vi "Turn_off_lamp.vi"() -> ()   [LabVIEW 2011]
uses:
  <vilib>/Instr/_visa.llb/VISA Configure Serial Port (Instr).vi
panel:
  in  "VISA resource name":refnum<visa-resource-name>="COM4"
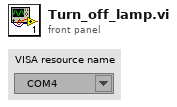
[diagram p1: front panel]
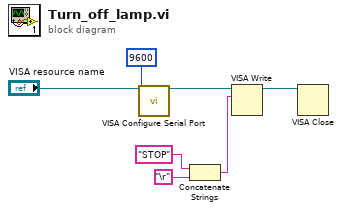
[diagram p0: block diagram]
diagram:
  n1 = call-poly "VISA Configure Serial Port"("VISA resource name"="VISA resource name", "baud rate (9600)"=u32 9600) -> ("VISA resource name out"=w5:refnum<visa-resource-name>)  [unwired: 12 in, 1 out]
  n2 = Concatenate Strings("STOP" ("write buffer"), "\r") -> (w2:string)
  n3 = VISA Write(VISA resource name=w5, write buffer=w2) -> (VISA resource name out=w1:refnum<visa-resource-name>)  [unwired: 1 in, 2 out]
  n4 = VISA Close(VISA resource name=w1) -> ()  [unwired: 1 in, 1 out]
